vi "Overview.vi"() -> ()   [LabVIEW 2024]
uses:
  <vilib>/Plug-In SDKs/Clients/Metadata/Operator.ctl
  <vilib>/Plug-In SDKs/Clients/Metadata/Extension.ctl
  <vilib>/Plug-In SDKs/Clients/Metadata/Test Station.ctl
  <vilib>/Plug-In SDKs/Clients/Metadata/Software Item.ctl
  <vilib>/Plug-In SDKs/Clients/Data Store V1/Data Store Client.lvlibp/API/Data Store V1/Test Result.ctl
  <vilib>/Plug-In SDKs/Clients/Metadata/Outcome.ctl
  <vilib>/Plug-In SDKs/Clients/Metadata/Step.ctl
  <vilib>/Plug-In SDKs/Clients/Metadata Store V1/Metadata Store Client.lvlibp/API/Metadata Store V1/Register Schema (Path).vi
  <vilib>/Plug-In SDKs/Clients/Metadata Store V1/Metadata Store Client.lvlibp/API/Metadata Store V1/Create Operator.vi
  <vilib>/Plug-In SDKs/Clients/Metadata Store V1/Metadata Store Client.lvlibp/API/Metadata Store V1/Create Test Station.vi
  <vilib>/Plug-In SDKs/Clients/Metadata Store V1/Metadata Store Client.lvlibp/API/Metadata Store V1/Create Software Item.vi
  <vilib>/Plug-In SDKs/Clients/Data Store V1/Data Store Client.lvlibp/API/Data Store V1/Publish Measurement (DBL Analog Waveform).vi
  <vilib>/Plug-In SDKs/Clients/Metadata Store V1/Metadata Store Client.lvlibp/API/Metadata Store V1/Get Operator.vi
  <vilib>/Plug-In SDKs/Clients/Data Store V1/Data Store Client.lvlibp/API/Data Store V1/Read Data from Measurement (DBL Analog Waveform).vi
  <vilib>/Plug-In SDKs/Clients/Metadata Store V1/Metadata Store Client.lvlibp
  <vilib>/Plug-In SDKs/Clients/Data Store V1/Data Store Client.lvlibp
  <vilib>/Plug-In SDKs/Clients/Metadata/NI Metadata Types.lvlib
  <vilib>/measure/NI_MABase.lvlib
panel:
  out "test result id":string
  out "published measurement id":string
  out "schema id":string
  out "queried data":waveform(dbl)(graph)
  out "log":string
  out "error out":errorcluster
  # "Overview\n\nThis example publishes a waveform along with metadata and extension attributes.\nThen it queries for the published data and displays it."
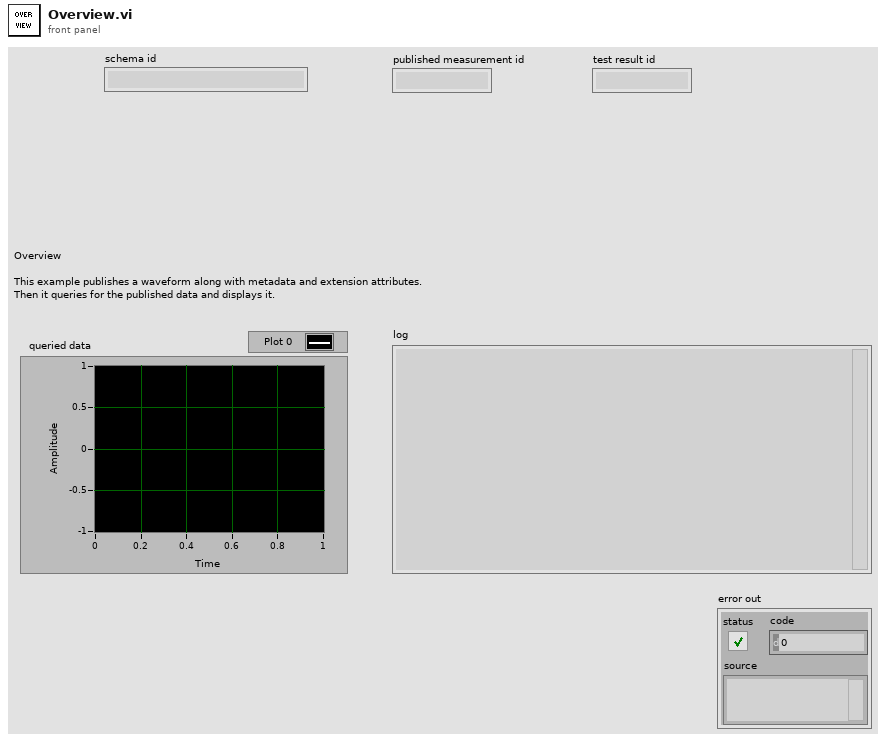
[diagram p1: front panel]
types:
  T1 = enum16{"Register Metadata Schema", "Create Metadata and Test Result", "Publish Data", "Query Published Data"}
  T2 = typedef "NI Metadata Types.lvlib/Extension.ctl" = cluster{"name":string, "value":string}
  T3 = typedef "Data Store Client.lvlibp/Test Result.ctl" = cluster{"test result name":string, "start date time":timestamp, "end date time":timestamp, "outcome":T4, "test result id":string, "uut instance id":string, "operator id":string, "test station id":string, "test description id":string, "software item ids":string[], "hardware item ids":string[], "test adapter ids":string[], "link":string, "extensions":T2[], "schema id":string}
  T4 = typedef "NI Metadata Types.lvlib/Outcome.ctl" = enum32{"Unspecified", "Passed", "Failed", "Indeterminate"}
  T5 = typedef "NI Metadata Types.lvlib/Software Item.ctl" = cluster{"product":string, "version":string, "id":string, "link":string, "extensions":T2[], "schema id":string}
  T6 = typedef "NI Metadata Types.lvlib/Test Station.ctl" = cluster{"test station name":string, "asset identifier":string, "id":string, "link":string, "extensions":T2[], "schema id":string}
  T7 = typedef "NI Metadata Types.lvlib/Operator.ctl" = cluster{"operator name":string, "role":string, "id":string, "link":string, "extensions":T2[], "schema id":string}
  T8 = typedef "NI Metadata Types.lvlib/Step.ctl" = cluster{"step name":string, "step type":string, "start date time":timestamp, "end date time":timestamp, "notes":string, "step id":string, "parent step id":string, "test result id":string, "test id":string, "link":string, "extensions":T2[], "schema id":string}
  T9 = typedef "Data Store Client.lvlibp/Published Measurement.ctl" = cluster{"data moniker":T10, "published conditions":T11[], "published measurement id":string, "test result id":string, "step id":string, "software item ids":string[], "hardware item ids":string[], "test adapter ids":string[], "measurement name":string, "data type":string, "measurement notes":string, "start date time":timestamp, "end date time":timestamp, "outcome":T4, "parametric index":i32, "error information":T12}
  T10 = typedef "Data Store Client.lvlibp/Data Moniker.ctl" = cluster{"service location":string, "data source":string, "data instance":i64}
  T11 = typedef "Data Store Client.lvlibp/Published Condition.ctl" = cluster{"moniker":T10, "published condition id":string, "condition name":string, "condition type":string, "step id":string, "test result id":string}
  T12 = typedef "NI Metadata Types.lvlib/Error Information.ctl" = cluster{"error code":i32, "message":string, "source":string}
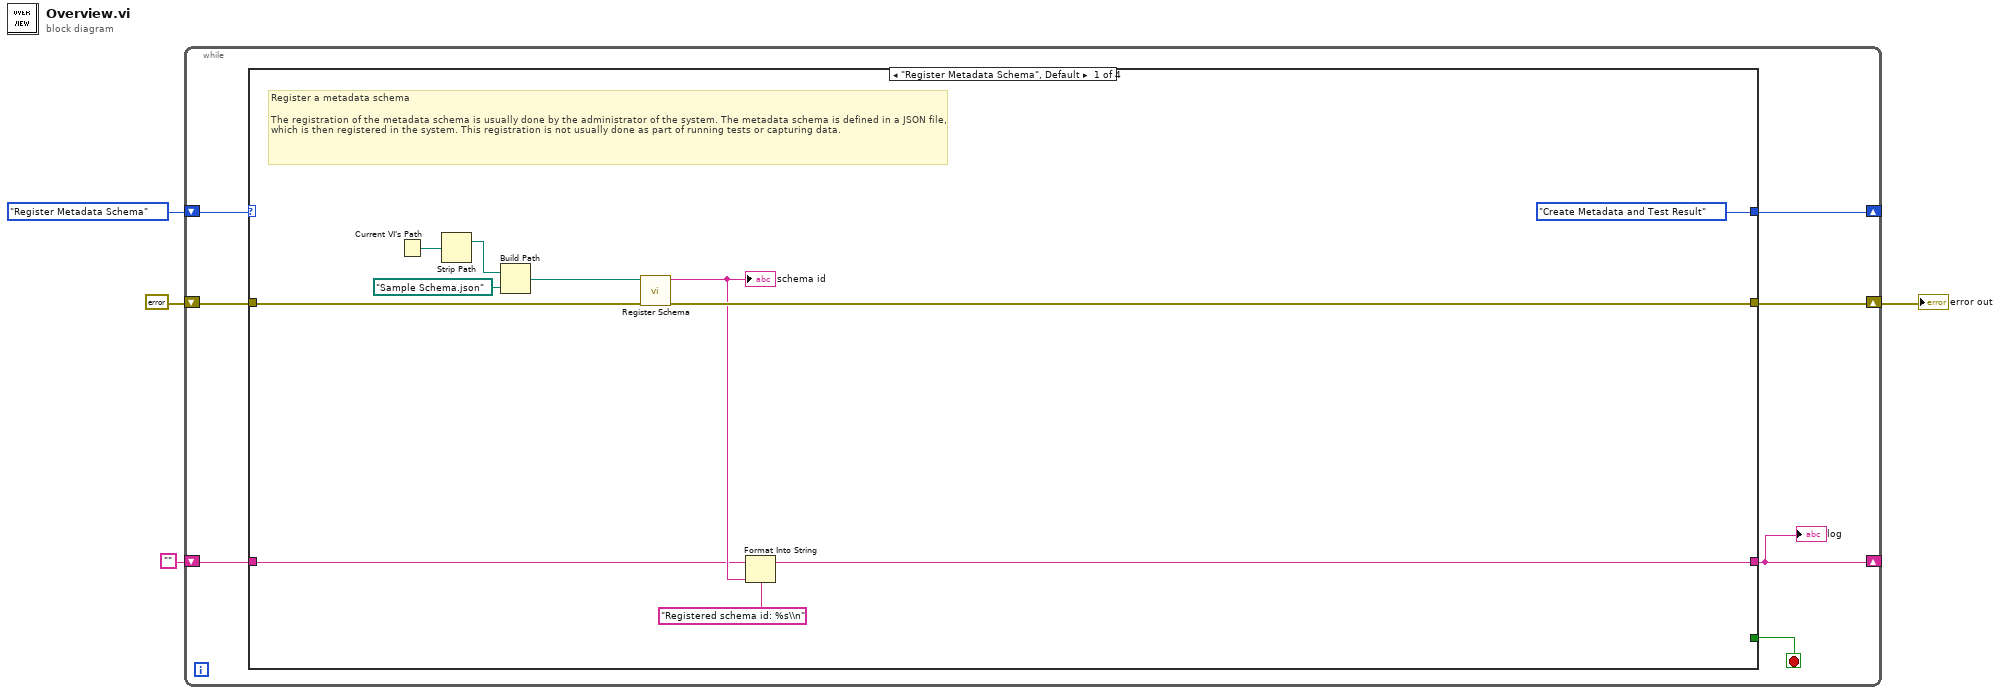
[diagram p0: block diagram]
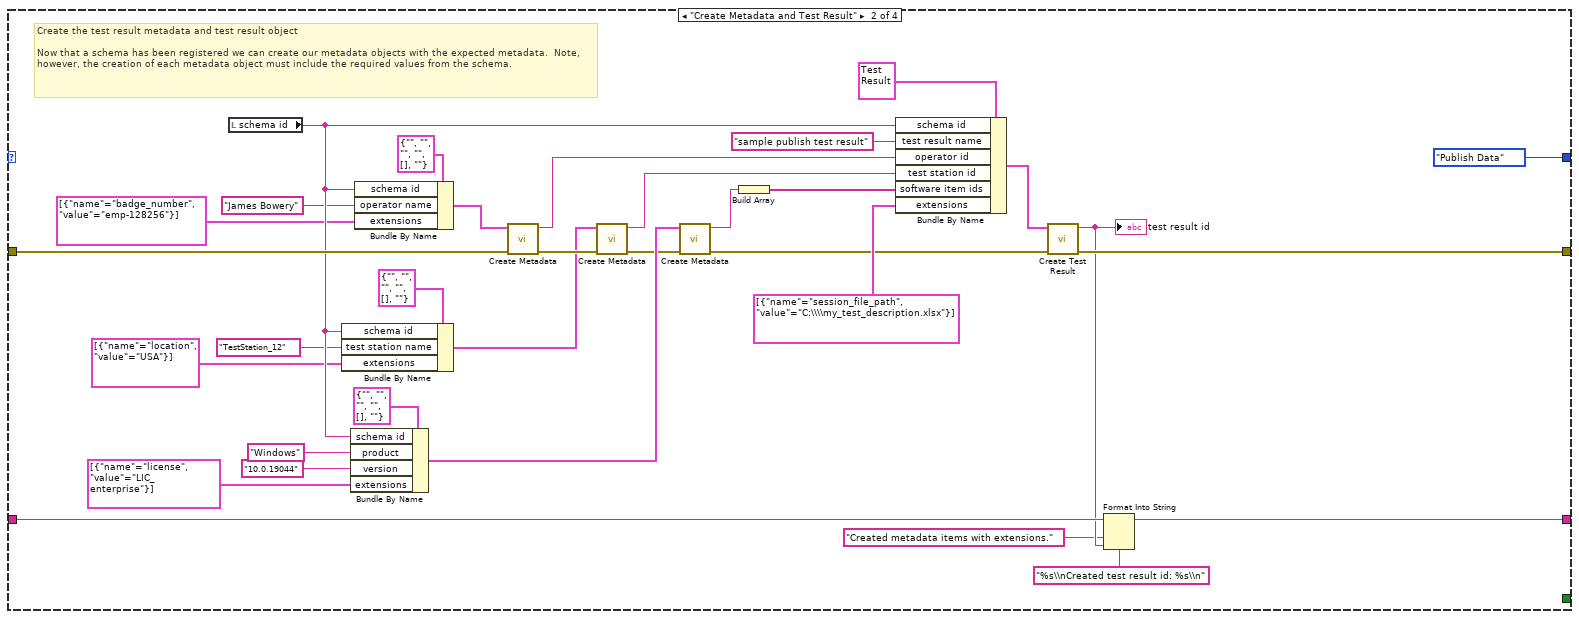
[diagram p2: hidden frame]
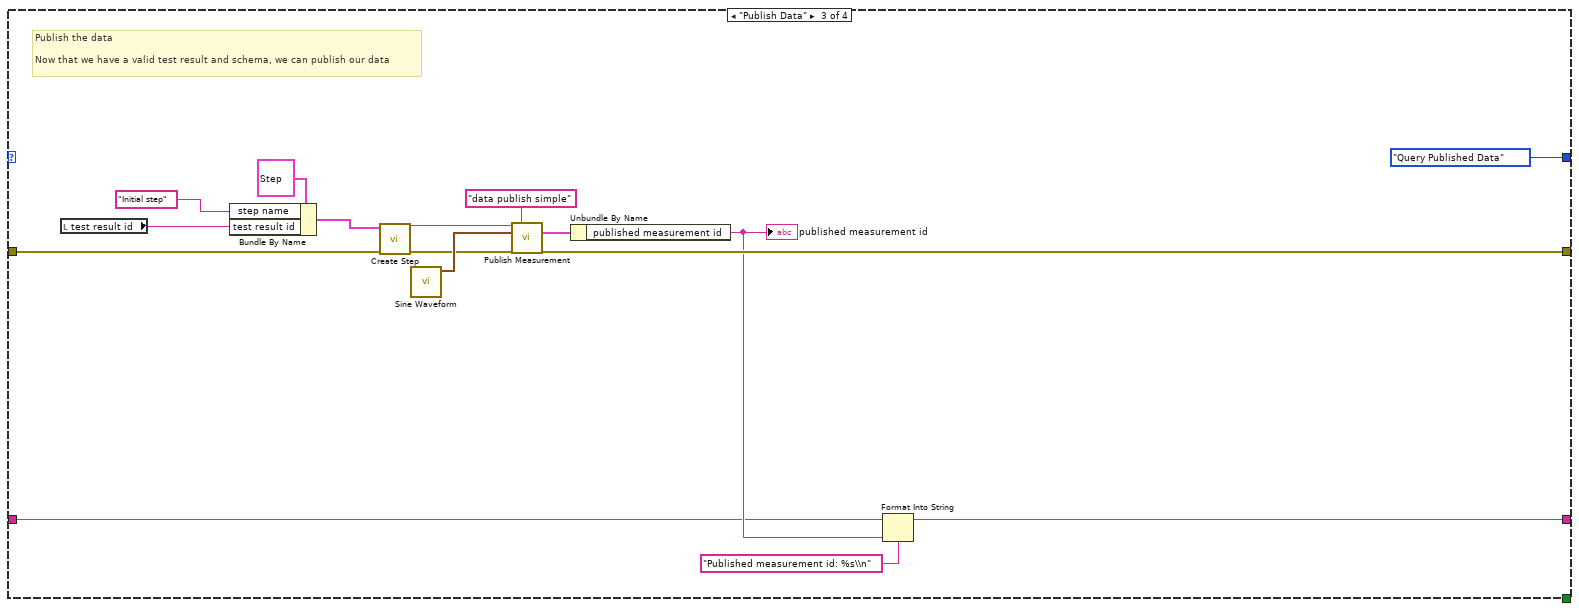
[diagram p3: hidden frame]
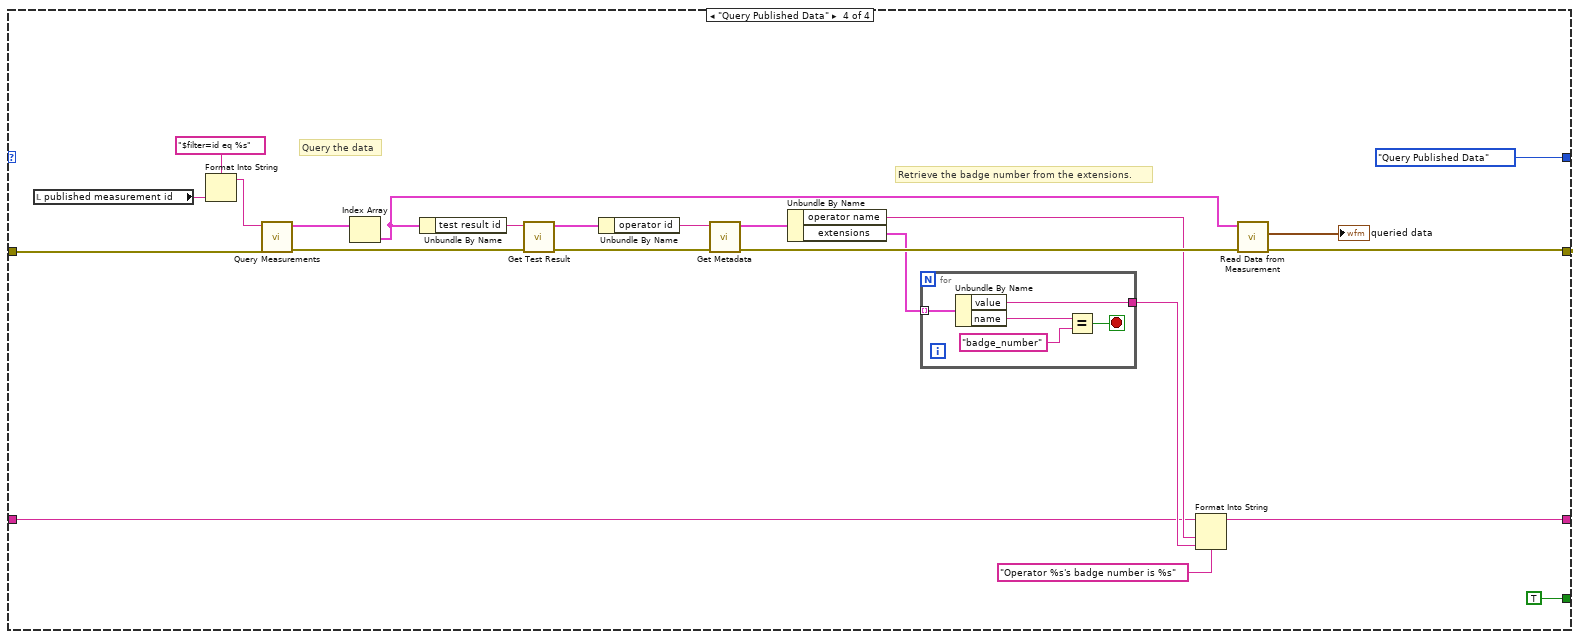
[diagram p4: hidden frame]
diagram:
  n1 = while {
    shift-right: [w7] -> _
    shift-left: T1."Register Metadata Schema" -> [w11]
    shift-right: [w10] -> w2
    shift-left: errorcluster {"status"=FALSE, "code"=0, "source"=""} ("error out") -> [w9]
    shift-right: [w6] -> _
    shift-left: "" ("log") -> [w8]
    stop <- w5 stop-if-true
    n2 = case shown="\"Register Metadata Schema\", Default" w11 {
      tunnel: [w22 w52 w71 w94] -> w10
      tunnel: w9 -> [w12 w53 w59 w93]
      tunnel: [w15 w49 w61 w73] -> w6
      tunnel: w8 -> [w16 w50 w56 w74]
      tunnel: [T1."Create Metadata and Test Result" T1."Publish Data" T1."Query Published Data" T1."Query Published Data"] -> w7
      tunnel: [_ _ _ TRUE] -> w5
      frame "Register Metadata Schema", Default {
        # "Register a metadata schema\n\nThe registration of the metadata schema is usually done by the administrator of the system. The metadata schema is defined in a JSON file, which is then registered in the system. This registration is not usually done as part of running tests or capturing data."
        n3 = Current VI's Path() -> (path=w19:path)
        n4 = Strip Path(path=w19) -> (stripped path=w18:path)  [unwired: 1 out]
        n5 = Build Path(base path=w18, name or relative path=path "Sample Schema.json") -> (appended path=w13:path)
        n6 = call-poly <vilib>:"Register Schema.vi"("error in"=w12, "schema"=w13) -> ("error out"=w22:errorcluster, "schema id"=w21:string)  [unwired: 8 in]
        "schema id" <- w21
        n7 = Format Into String(format string="Registered schema id: %s\\n", initial string=w16, w21) -> (resulting string=w15:string)  [unwired: 1 in, 1 out]
      }
      frame "Create Metadata and Test Result" {
        # "Create the test result metadata and test result object\n\nNow that a schema has been registered we can create our metadata objects with the expected metadata.  Note, however, the creation of each metadata object must include the required values from the schema."
        n8 = local read "schema id"() -> (w51:string)
        n9 = Bundle By Name(cluster=T6 {"test station name"="", "asset identifier"="", "id"="", "link"="", "extensions"=[], "schema id"=""} ("test station"), "schema id"=w51, "test station name"="TestStation_12", "extensions"=T2[] [{"name"="location", "value"="USA"}]) -> (w23:T6)
        n10 = Bundle By Name(cluster=T5 {"product"="", "version"="", "id"="", "link"="", "extensions"=[], "schema id"=""} ("software item"), "schema id"=w51, "product"="Windows", "version"="10.0.19044", "extensions"=T2[] [{"name"="license", "value"="LIC_enterprise"}]) -> (w27:T5)
        n11 = Bundle By Name(cluster=T7 {"operator name"="", "role"="", "id"="", "link"="", "extensions"=[], "schema id"=""} ("operator metadata"), "schema id"=w51, "operator name"="James Bowery", "extensions"=T2[] [{"name"="badge_number", "value"="emp-128256"}]) -> (w34:T7)
        n12 = call-poly <vilib>:"Create Metadata.vi"("error in"=w53, "operator metadata"=w34) -> ("error out"=w26:errorcluster, "operator id"=w45:string)  [unwired: 8 in]
        n13 = call-poly <vilib>:"Create Metadata.vi"("error in"=w26, "test station"=w23) -> ("error out"=w25:errorcluster, "test station id"=w44:string)  [unwired: 8 in]
        n14 = call-poly <vilib>:"Create Metadata.vi"("error in"=w25, "software item"=w27) -> ("error out"=w24:errorcluster, "software item id"=w43:string)  [unwired: 8 in]
        n15 = Build Array(w43) -> (w40:string[])
        n16 = Bundle By Name(cluster=T3 {"test result name"="", "start date time"=timestamp(0 s since 1904-01-01), "end date time"=timestamp(0 s since 1904-01-01), "outcome"=enum."Unspecified", "test result id"="", "uut instance id"="", "operator id"="", "test station id"="", "test description id"="", "software item ids"=[], "hardware item ids"=[], "test adapter ids"=[], "link"="", "extensions"=[], "schema id"=""} ("test result"), "schema id"=w51, "test result name"="sample publish test result", "operator id"=w45, "test station id"=w44, "software item ids"=w40, "extensions"=T2[] [{"name"="session_file_path", "value"="C:\\\\my_test_description.xlsx"}]) -> (w55:T3)
        n17 = call <vilib>:"Create Test Result.vi"("error in"=w24, "test result"=w55) -> ("error out"=w52:errorcluster, "test result id"=w47:string)  [unwired: 8 in]
        "test result id" <- w47
        n18 = Format Into String(format string="%s\\nCreated test result id: %s\\n", initial string=w50, "Created metadata items with extensions." ("log"), w47) -> (resulting string=w49:string)  [unwired: 1 in, 1 out]
      }
      frame "Publish Data" {
        # "Publish the data\n\nNow that we have a valid test result and schema, we can publish our data"
        n19 = local read "test result id"() -> (w58:string)
        n20 = Bundle By Name(cluster=T8 {"step name"="", "step type"="", "start date time"=timestamp(0 s since 1904-01-01), "end date time"=timestamp(0 s since 1904-01-01), "notes"="", "step id"="", "parent step id"="", "test result id"="", "test id"="", "link"="", "extensions"=[], "schema id"=""} ("step"), "step name"="Initial step", "test result id"=w58) -> (w66:T8)
        n21 = call <vilib>:"Create Step.vi"("error in"=w59, "step"=w66) -> ("error out"=w65:errorcluster, "step id"=w64:string)  [unwired: 8 in]
        n22 = call <vilib>:"Sine Waveform.vi"() -> ("signal out"=w69:waveform(dbl))  [unwired: 10 in, 1 out]
        n23 = call-poly <vilib>:"Publish Measurement.vi"("step id"=w64, "name"="data publish simple", "waveform"=w69, "error in"=w65) -> ("published measurement"=w62:T9, "error out"=w71:errorcluster)  [unwired: 9 in, 1 out]
        n24 = Unbundle By Name(w62) -> ("published measurement id"=w70:string)
        "published measurement id" <- w70
        n25 = Format Into String(format string="Published measurement id: %s\\n", initial string=w56, w70) -> (resulting string=w61:string)  [unwired: 1 in, 1 out]
      }
      frame "Query Published Data" {
        # "Retrieve the badge number from the extensions."
        # "Query the data"
        n26 = local read "published measurement id"() -> (w92:string)
        n27 = Format Into String(format string="$filter=id eq %s", w92) -> (resulting string=w83:string)  [unwired: 2 in, 1 out]
        n28 = call <vilib>:"Query Measurements.vi"("error in"=w93, "odata query"=w83) -> ("error out"=w81:errorcluster, "published measurements"=w82:T9[])  [unwired: 8 in]
        n29 = Index Array(array=w82) -> (element=w75:T9)  [unwired: 1 in]
        n30 = Unbundle By Name(w75) -> ("test result id"=w80:string)
        n31 = call <vilib>:"Get Test Result.vi"("error in"=w81, "test result id"=w80) -> ("error out"=w79:errorcluster, "test result"=w78:T3)  [unwired: 8 in]
        n32 = Unbundle By Name(w78) -> ("operator id"=w77:string)
        n33 = call-poly <vilib>:"Get Metadata.vi"("error in"=w79, "operator id"=w77) -> ("error out"=w89:errorcluster, "operator metadata"=w76:T7)  [unwired: 8 in]
        n34 = Unbundle By Name(w76) -> ("operator name"=w86:string, "extensions"=w87:T2[])
        n35 = for {
          tunnel: w87 -> [w99] mode=indexing
          tunnel: [w95] -> w88
          stop <- w96 stop-if-true
          n36 = Unbundle By Name(w99) -> ("value"=w95:string, "name"=w98:string)
          n37 = Equal?(x=w98, y="badge_number") -> (x = y?=w96:bool)
        }
        n38 = Format Into String(format string="Operator %s's badge number is %s", initial string=w74, w86, w88) -> (resulting string=w73:string)  [unwired: 1 in, 1 out]
        n39 = call-poly <vilib>:"Read Data from Measurement.vi"("error in"=w89, "published measurement"=w75) -> ("error out"=w94:errorcluster, "waveform data"=→"queried data":waveform(dbl))  [unwired: 7 in, 1 out]
      }
    }
    "log" <- w6
  }
  "error out" <- w2
